vi "NO calc loffPIDA.vi"(4 "I":dbl, 6 "Feed":dbl, 7 "P":dbl, 8 "Flow Rate":dbl, 9 "NOm ppm":dbl, 10 "NO Conc":dbl, 11 "NOt ppm":dbl) -> (2 "NO MFR":dbl)   [LabVIEW 2011]
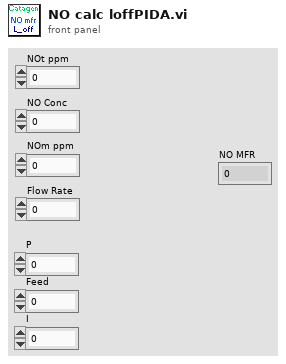
[diagram p1: front panel]
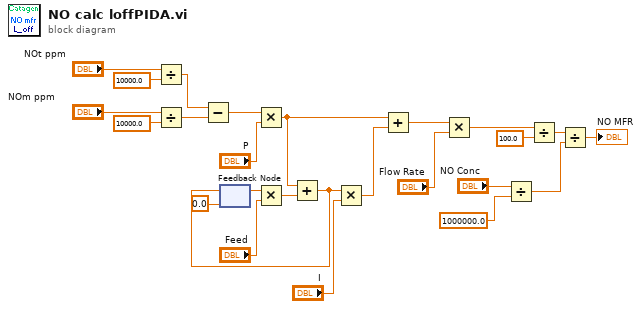
[diagram p0: block diagram]
diagram:
  n1 = Divide(x="NOt ppm", y=10000.0) -> (x/y=w14:dbl)
  n2 = Divide(x="NOm ppm", y=10000.0) -> (x/y=w15:dbl)
  n3 = Subtract(x=w14, y=w15) -> (x-y=w13:dbl)
  n4 = feedback #1(0.0) -> (w6:dbl)
  n5 = Multiply(x=w13, y="P") -> (x*y=w11:dbl)
  n6 = Multiply(x=w6, y="Feed") -> (x*y=w5:dbl)
  n7 = Add(x=w11, y=w5) -> (x+y=w7:dbl)
  n8 = feedback-in #1(w7) -> ()
  n9 = Multiply(x=w7, y="I") -> (x*y=w10:dbl)
  n10 = Add(x=w11, y=w10) -> (x+y=w9:dbl)
  n11 = Multiply(x=w9, y="Flow Rate") -> (x*y=w20:dbl)
  n12 = Divide(x="NO Conc", y=1000000.0) -> (x/y=w16:dbl)
  n13 = Divide(x=w20, y=100.0) -> (x/y=w19:dbl)
  n14 = Divide(x=w19, y=w16) -> (x/y=→"NO MFR":dbl)
